vi "practica3.vi"() -> ()   [LabVIEW 2018]
panel:
  in  "PUERTO USB":refnum<visa-resource-name>
  in  "stop":bool
  in  "CONTROL RGB":enum32{"Page 1", "Page 2"}(tab)
  in  "OK Button 2":bool
  out "Sin campo magnetico":bool
  out "Con campo magnetico":bool
  in  "OK Button":bool
  in  "Puerto entrada Hall":dbl
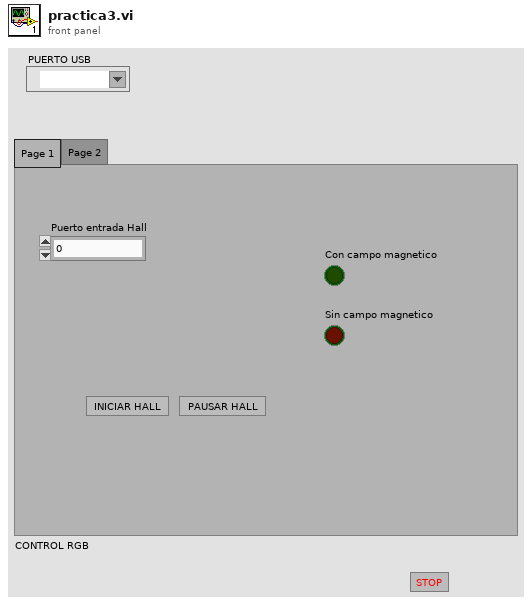
[diagram p1: front panel]
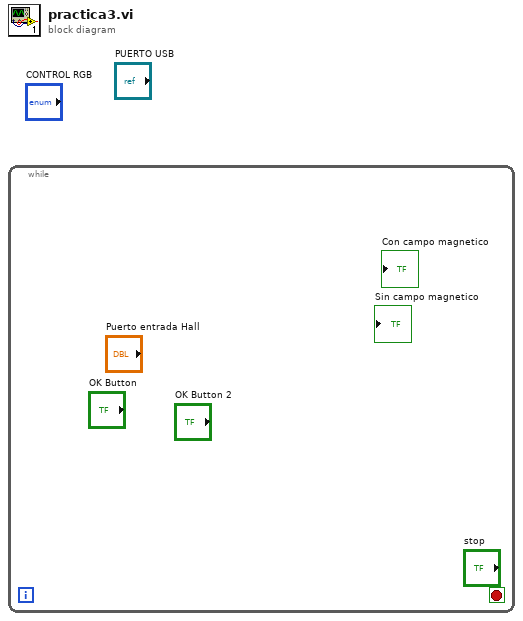
[diagram p0: block diagram]
diagram:
  n1 = while {
    stop <- _ stop-if-true
  }
